vi "WPI_Power Get Rail Voltage and Current.vi"   [LabVIEW 2017]
doc: "Returns the voltage and current of a user rail on the roboRIO."
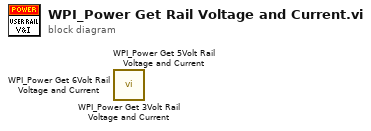
[diagram p0: block diagram]
diagram:
  n1 = call <vilib>:"WPI_Power Get 3Volt Rail Voltage and Current.vi"() -> ()  [unwired: 13 in, 3 out]
  n2 = call <vilib>:"WPI_Power Get 5Volt Rail Voltage and Current.vi"() -> ()  [unwired: 13 in, 3 out]
  n3 = call <vilib>:"WPI_Power Get 6Volt Rail Voltage and Current.vi"() -> ()  [unwired: 13 in, 3 out]
